vi "Esophageal_Datalogger_SaveButton.vi"(6 "HRME Score":string="Auto Gain Selected", 8 "error in (no error)":errorcluster, 9 "Timestamp":string="Auto Gain Selected", 10 "Image Name":string="Auto Gain Selected", 11 "Log File In":refnum<file>) -> (0 "error out":errorcluster, 3 "Log File Out":refnum<file>)   [LabVIEW 2021]
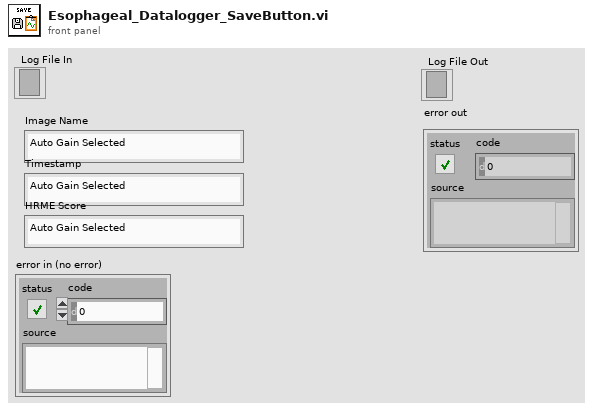
[diagram p1: front panel]
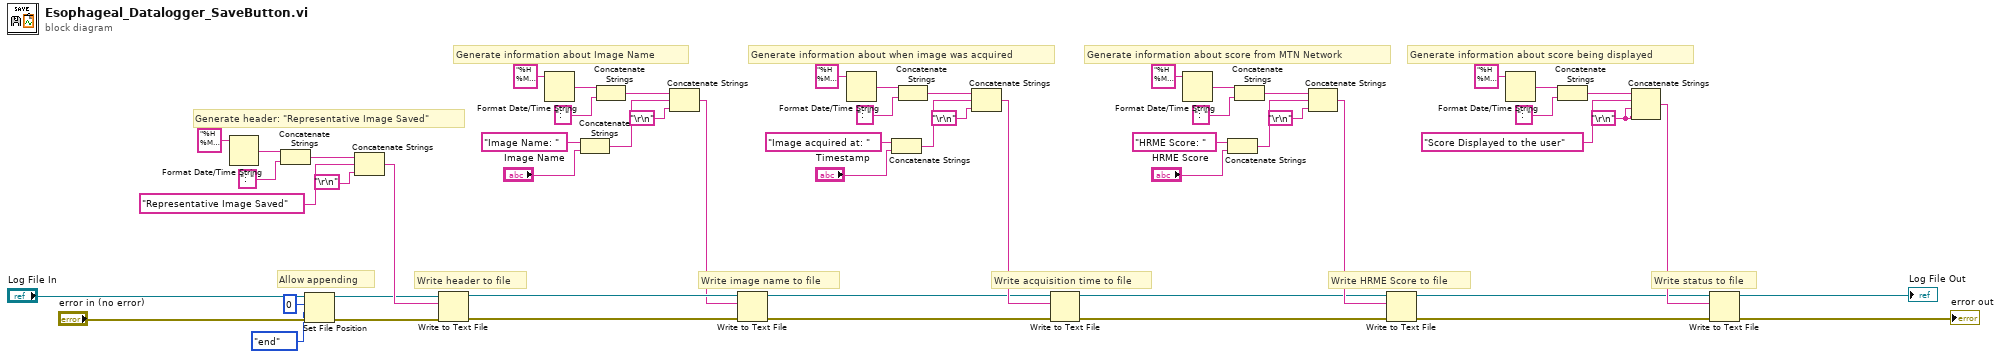
[diagram p0: block diagram]
diagram:
  w2 = "\r\n"
  # "Generate information about score being displayed"
  # "Write status to file"
  # "Generate information about score from MTN Network"
  # "Write HRME Score to file"
  # "Generate information about when image was acquired"
  # "Generate information about Image Name"
  # "Write image name to file"
  # "Write header to file"
  # "Generate header: \"Representative Image Saved\""
  # "Write acquisition time to file"
  # "Allow appending"
  n1 = Format Date/Time String(time format string (%c)="%H%M%S%3u") -> (date/time string=w36:string)  [unwired: 2 in]
  n2 = Concatenate Strings(w36, ": " ("string")) -> (w38:string)
  n3 = Set File Position(offset (in bytes) (0)=i64 0, refnum="Log File In", from (0:start)=enum16{"start", "end", "current"}."end", error in="error in (no error)") -> (refnum out=w34:refnum<file>, error out=w42:errorcluster)
  n4 = Concatenate Strings(w38, "Representative Image Saved" ("time format string (%c)"), "\r\n") -> (w41:string)
  n5 = Write to Text File(file (use dialog)=w34, text=w41, error in=w42) -> (refnum out=w49:refnum<file>, error out=w50:errorcluster)  [unwired: 1 in, 1 out]
  n6 = Format Date/Time String(time format string (%c)="%H%M%S%3u") -> (date/time string=w46:string)  [unwired: 2 in]
  n7 = Concatenate Strings("Image Name: " ("time format string (%c)"), "Image Name") -> (w27:string)
  n8 = Concatenate Strings(w46, ": " ("string")) -> (w44:string)
  n9 = Concatenate Strings(w44, w27, "\r\n") -> (w48:string)
  n10 = Write to Text File(file (use dialog)=w49, text=w48, error in=w50) -> (refnum out=w51:refnum<file>, error out=w52:errorcluster)  [unwired: 1 in, 1 out]
  n11 = Format Date/Time String(time format string (%c)="%H%M%S%3u") -> (date/time string=w54:string)  [unwired: 2 in]
  n12 = Concatenate Strings("Image acquired at: " ("time format string (%c)"), "Timestamp") -> (w24:string)
  n13 = Concatenate Strings(w54, ": " ("string")) -> (w56:string)
  n14 = Concatenate Strings(w56, w24, "\r\n") -> (w57:string)
  n15 = Write to Text File(file (use dialog)=w51, text=w57, error in=w52) -> (refnum out=w13:refnum<file>, error out=w12:errorcluster)  [unwired: 1 in, 1 out]
  n16 = Format Date/Time String(time format string (%c)="%H%M%S%3u") -> (date/time string=w17:string)  [unwired: 2 in]
  n17 = Concatenate Strings("HRME Score: " ("time format string (%c)"), "HRME Score") -> (w21:string)
  n18 = Concatenate Strings(w17, ": " ("string")) -> (w15:string)
  n19 = Concatenate Strings(w15, w21, "\r\n") -> (w14:string)
  n20 = Write to Text File(file (use dialog)=w13, text=w14, error in=w12) -> (refnum out=w6:refnum<file>, error out=w5:errorcluster)  [unwired: 1 in, 1 out]
  n21 = Format Date/Time String(time format string (%c)="%H%M%S%3u") -> (date/time string=w8:string)  [unwired: 2 in]
  n22 = Concatenate Strings(w8, ": " ("string")) -> (w10:string)
  n23 = Concatenate Strings(w10, "Score Displayed to the user" ("time format string (%c)"), w2, w2) -> (w11:string)
  n24 = Write to Text File(file (use dialog)=w6, text=w11, error in=w5) -> (refnum out=→"Log File Out":refnum<file>, error out=→"error out":errorcluster)  [unwired: 1 in, 1 out]
